vi "更新易损件.vi"(8 "error in (no error)":errorcluster caption="错误输入（无错误）") -> (0 "error out":errorcluster)   [LabVIEW 2018]
uses:
  <vilib>/addons/database/Connection.llb/DB Tools Open Connec (String).vi
  <vilib>/addons/database/Connection.llb/Conn Execute.vi
  <vilib>/addons/database/Recordset.llb/Rec Fetch Recordset Data (R).vi
  <vilib>/addons/database/Recordset.llb/Rec Destroy - Connection.vi
  <vilib>/addons/database/NI_Database_API.lvlib
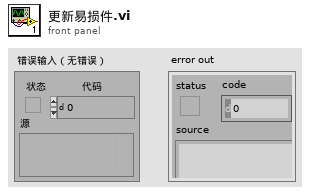
[diagram p1: front panel]
types:
  T1 = typedef "NI_Database_API.lvlib/Conn ObjectReference.ctl" = refnum<k1>
  T2 = typedef "NI_Database_API.lvlib/Rec ObjectReference.ctl" = refnum<k1>
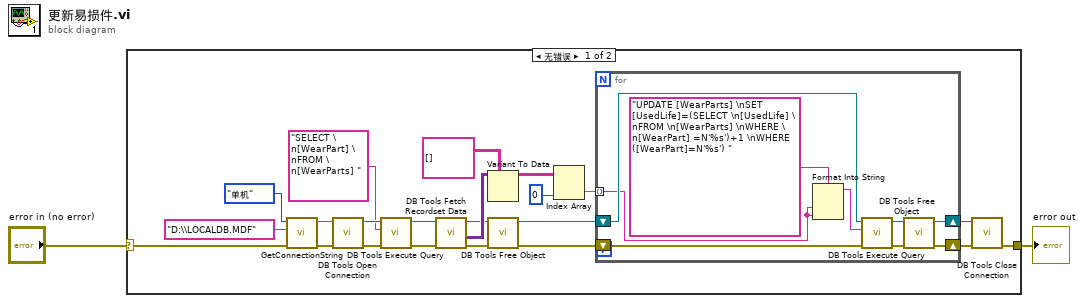
[diagram p0: block diagram]
diagram:
  n1 = case shown="无错误" "error in (no error)" {
    selector: "error in (no error)" -> [w3 w34]
    tunnel: [w17 w34] -> w2
    frame No Error {
      n2 = call "GetConnectionString.vi"("error in (no error)"=w3, "Database Name"="D:\\LOCALDB.MDF", "连接模式"=enum16{"单机", "联网"}."单机") -> ("error out"=w23:errorcluster, "连接字符串"=w22:string)  [unwired: 3 in]
      n3 = call-poly <vilib>:"DB Tools Open Connection.vi"("error in (no error)"=w23, "connection information"=w22) -> ("error out"=w21:errorcluster, "connection reference"=w20:T1)  [unwired: 6 in]
      n4 = call-poly <vilib>:"DB Tools Execute Query.vi"("error in (no error)"=w21, "SQL query"="SELECT \n[WearPart] \nFROM \n[WearParts] ", "connection reference"=w20) -> ("error out"=w15:errorcluster, "recordset reference"=w14:T2)  [unwired: 5 in]
      n5 = call-poly <vilib>:"DB Tools Fetch Recordset Data.vi"("error in (no error)"=w15, "recordset reference"=w14) -> ("error out"=w8:errorcluster, "recordset data"=w13:variant[][], "recordset reference out"=w9:T2)  [unwired: 3 in]
      n6 = Variant To Data(type=string[][] [], Variant=w13) -> (data=w11:string[][])  [unwired: 1 in, 1 out]
      n7 = call-poly <vilib>:"DB Tools Free Object.vi"("error in (no error)"=w8, "recordset reference"=w9) -> ("error out"=w6:errorcluster, "connection reference"=w7:T1)  [unwired: 8 in]
      n8 = Index Array(array=w11, index (col)=0 ("禁用的索引 (列)")) -> (element=w5:string[])  [unwired: 1 in]
      n9 = for {
        shift-right: [w32] -> w18
        shift-left: w7 -> [w28]
        shift-right: [w33] -> w19
        shift-left: w6 -> [w27]
        tunnel: w5 -> [w26] mode=indexing
        n10 = Format Into String(format string="UPDATE [WearParts] \nSET [UsedLife]=(SELECT \n[UsedLife] \nFROM \n[WearParts] \nWHERE \n[WearPart] =N'%s')+1 \nWHERE ([WearPart]=N'%s') " ("格式字符串"), w26, w26) -> (resulting string=w25:string)  [unwired: 2 in, 1 out]
        n11 = call-poly <vilib>:"DB Tools Execute Query.vi"("error in (no error)"=w27, "SQL query"=w25, "connection reference"=w28) -> ("error out"=w29:errorcluster, "recordset reference"=w30:T2)  [unwired: 5 in]
        n12 = call-poly <vilib>:"DB Tools Free Object.vi"("error in (no error)"=w29, "recordset reference"=w30) -> ("error out"=w33:errorcluster, "connection reference"=w32:T1)  [unwired: 8 in]
      }
      n13 = call <vilib>:"DB Tools Close Connection.vi"("error in (no error)"=w19, "connection reference"=w18) -> ("error out"=w17:errorcluster)  [unwired: 5 in]
    }
    frame Error {
    }
  }
  "error out" <- w2
